vi "Variable Length FIFO-write.vi"(8 "error in (no error)":errorcluster, 10 "DAQ Input Parameters(FlexRIO)":T1 {"diff_threshZ" format="%#_11g"; "proportioanl_scale Z" format="%#_15g"; "var_x" format="%#_14g"; "var_y" format="%#_14g"; "scale" format="%#_15g"; "diff_thresh" format="%#_11g"; "proportioanl_scale" format="%#_15g"}, 11 "FGPA Ref":T4) -> (0 "error out":errorcluster, 3 "FGPA Ref":T4)   [LabVIEW 2020]
uses:
  <vilib>/rvi/interface/nirviMethod/nirviMethod.xnode
  RIG-SPECIFIC FILES/FPGA Refs/FPGA Ref.ctl
  <vilib>/rvi/errors/niLvFpgaMergeErrorWithErrorCode.vi
  <vilib>/FPGAPlugInAG/Dynamic/niLvFpga_StopFifo_Dynamic.vi
  <vilib>/FPGAPlugInAG/Dynamic/niLvFpga_StartFifo_Dynamic.vi
  <vilib>/FPGAPlugInAG/Dynamic/niLvFpga_WriteFifo_Dynamic.vi
  FPGA Host VIs/typedefs/scan_type.ctl
  Movement Correction/Typedefs/Control algorithm.ctl
  Typedefs/Controls/DAQ Input Parameters(FlexRIO).ctl
panel:
  out "Empty Elements Remaining":u32
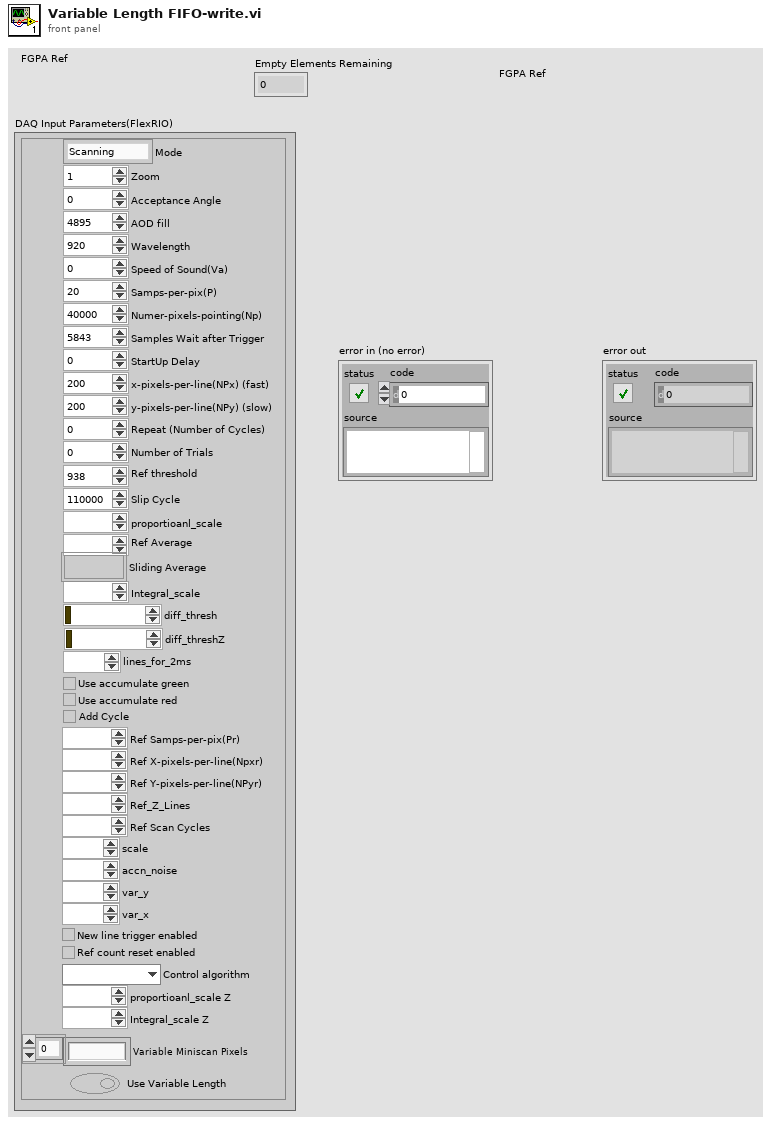
[diagram p1: front panel]
types:
  T1 = typedef "DAQ Input Parameters(FlexRIO).ctl" = cluster{"Mode":T2, "Zoom":i8, "Acceptance Angle":i8, "AOD fill":u16, "Wavelength":i16, "Speed of Sound(Va)":i8, "Samps-per-pix(P)":i16, "Numer-pixels-pointing(Np)":u32, "Samples Wait after Trigger":u16, "StartUp Delay":i32, "x-pixels-per-line(NPx) (fast)":u16, "y-pixels-per-line(NPy) (slow)":u16, "Repeat (Number of Cycles)":u32, "Number of Trials":u16, "Ref threshold":u16, "Slip Cycle":u32, "proportioanl_scale":fxp<+,16,2>, "Ref Average":u16, "Sliding Average":bool, "Integral_scale":fxp<+/-,16,12>, "diff_thresh":fxp<+/-,16,8>, "diff_threshZ":fxp<+/-,16,8>, "lines_for_2ms":i16, "Use accumulate green":bool, "Use accumulate red":bool, "Add Cycle":bool, "Ref Samps-per-pix(Pr)":i16, "Ref X-pixels-per-line(Npxr)":i16, "Ref Y-pixels-per-line(NPyr)":i16, "Ref_Z_Lines":i16, "Ref Scan Cycles":i32, "scale":fxp<+,16,2>, "accn_noise":fxp<+,16,16>, "var_y":fxp<+,16,4>, "var_x":fxp<+,16,4>, "New line trigger enabled":bool, "Ref count reset enabled":bool, "Control algorithm":T3, "proportioanl_scale Z":fxp<+,16,2>, "Integral_scale Z":fxp<+/-,16,12>, "Variable Miniscan Pixels":u16[], "Use Variable Length":bool}
  T2 = typedef "scan_type.ctl" = enum16{"Scanning", "Pointing", "Pointing & MC", "Scanning & MC"}
  T3 = typedef "Control algorithm.ctl" = enum16{"PID", "Kalman"}
  T4 = typedef "FPGA Ref.ctl" = refnum<k20>
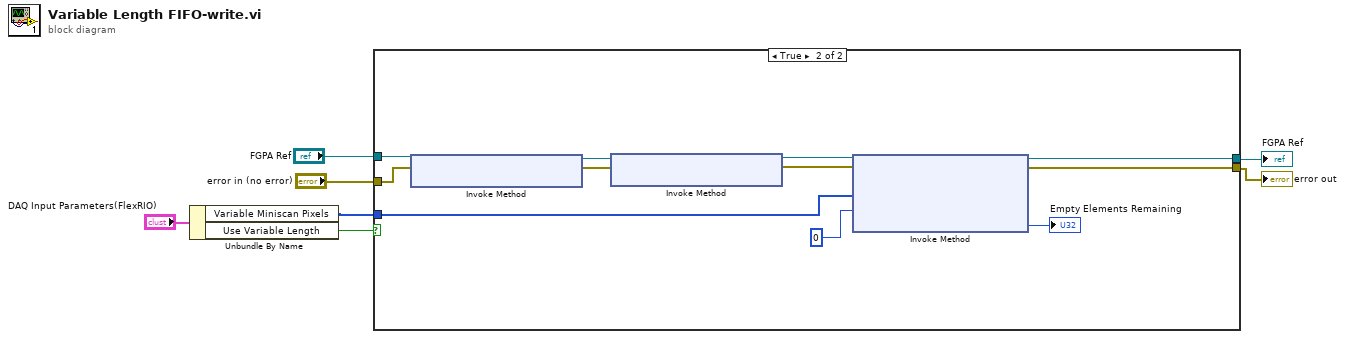
[diagram p0: block diagram]
diagram:
  n1 = Unbundle By Name("DAQ Input Parameters(FlexRIO)") -> ("Variable Miniscan Pixels"=w2:u16[], "Use Variable Length"=w1:bool)
  n2 = case shown="True" w1 {
    tunnel: "FGPA Ref" -> [w9 w16]
    tunnel: [w9 w20] -> w6
    tunnel: "error in (no error)" -> [w8 w15]
    tunnel: [w8 w19] -> w4
    tunnel: w2 -> [_ w17]
    frame False {
    }
    frame True {
      n3 = xnode "Invoke Method"("FPGA VI Reference In"=w16, "error in"=w15) -> ("FPGA VI Reference Out"=w13:T4, "error out"=w12:errorcluster)
      n4 = xnode "Invoke Method"("FPGA VI Reference In"=w13, "error in"=w12) -> ("FPGA VI Reference Out"=w10:T4, "error out"=w11:errorcluster)
      n5 = xnode "Invoke Method"("FPGA VI Reference In"=w10, "error in"=w11, "Data"=w17, "Timeout (ms)"=0) -> ("FPGA VI Reference Out"=w20:T4, "error out"=w19:errorcluster, "Empty Elements Remaining"=→"Empty Elements Remaining":u32)
    }
  }
  "FGPA Ref" <- w6
  "error out" <- w4
